vi "Error - Fire.vi"(6 "Source":variant, 7 "Date Time":string, 8 "error in (no error)":errorcluster, 9 "Description":string, 10 "Error Type":T1, 11 "View Model":T2) -> (0 "error out":errorcluster, 3 "View Model":T2)   [LabVIEW 2017]
doc: "Generates Error user event with addiditonal parameters."
uses:
  View Model/Controls/View Model.ctl
  View Model/Controls/Shared Model.ctl
  Controls/Error Model.ctl
  Controls/Error Event.ctl
  Controls/Error Type.ctl
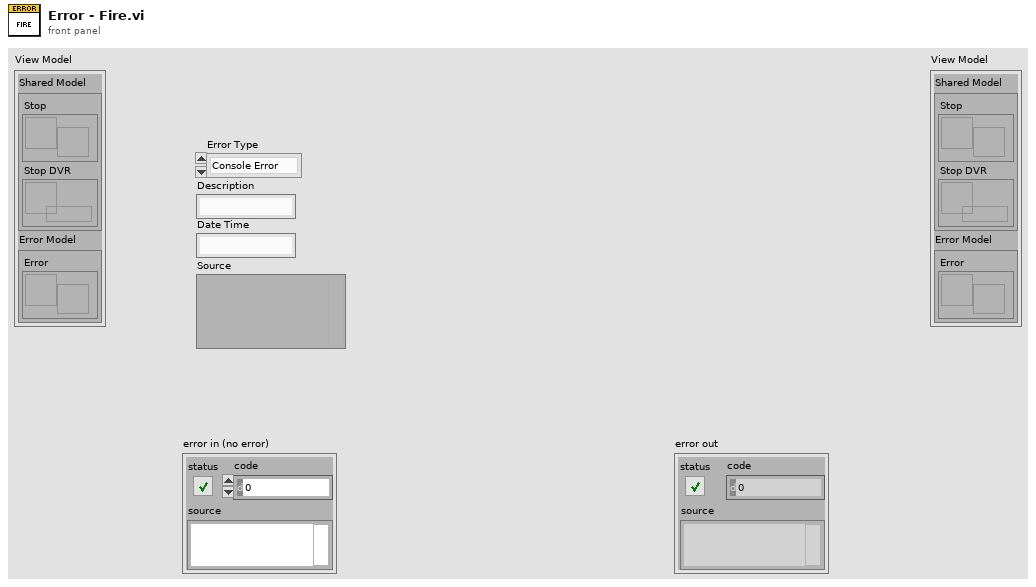
[diagram p1: front panel]
types:
  T1 = typedef "Error Type.ctl" = enum16{"Console Error", "Sensor Interface IO Error", "Process Step Error"}
  T2 = typedef "View Model.ctl" = cluster{"Shared Model":T3, "Error Model":T4}
  T3 = typedef "Shared Model.ctl" = cluster{"Stop":refnum<user-event>, "Stop DVR":refnum<data-value>}
  T4 = typedef "Error Model.ctl" = cluster{"Error":refnum<user-event>}
  T5 = typedef "Error Event.ctl" = cluster{"Error Type":T1, "Description":string, "Date Time":string, "Source":variant}
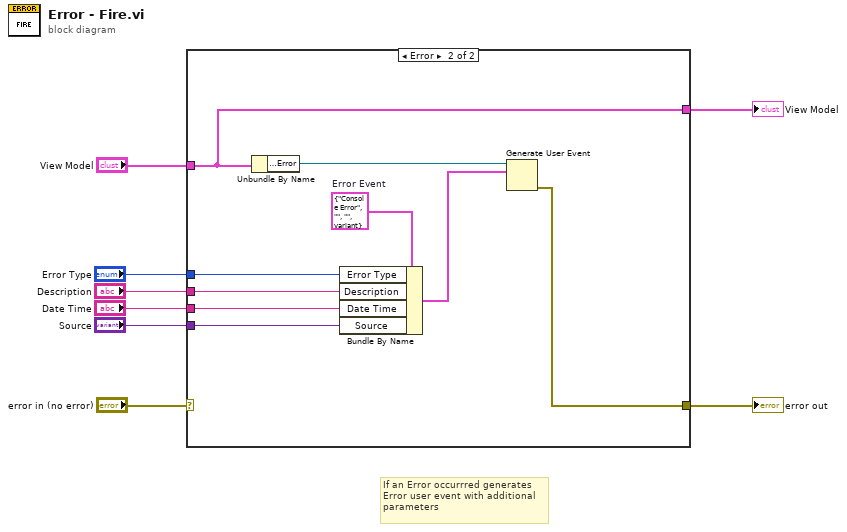
[diagram p0: block diagram]
diagram:
  # "If an Error occurrred generates\nError user event with additional\nparameters"
  n1 = case shown="Error" "error in (no error)" {
    selector: "error in (no error)" -> [w9 _]
    tunnel: "View Model" -> [w10 w11]
    tunnel: [w10 w11] -> w6
    tunnel: [w9 w12] -> w5
    tunnel: "Source" -> [_ w17]
    tunnel: "Date Time" -> [_ w16]
    tunnel: "Description" -> [_ w15]
    tunnel: "Error Type" -> [_ w14]
    frame No Error {
    }
    frame Error {
      w18 = T5 {"Error Type"=enum."Console Error", "Description"="", "Date Time"="", "Source"=variant}  # Error Event
      n2 = Unbundle By Name(w11) -> ("Error Model.Error"=w19:refnum<user-event>)
      n3 = Bundle By Name(cluster=w18, "Error Type"=w14, "Description"=w15, "Date Time"=w16, "Source"=w17) -> (w13:T5)
      n4 = Generate User Event(user event=w19, event data cluster=w13) -> (error out=w12:errorcluster)  [unwired: 2 in, 1 out]
    }
  }
  "error out" <- w5
  "View Model" <- w6
